vi "UtilityLib.Sixcolor.vi"(0 "State":T1 caption="index") -> (3 "booleanColor":u32(colorbox), 4 "elementBackground":u32(colorbox), 5 "elementText":u32(colorbox), 6 "elementTextWhite":u32(colorbox))   [LabVIEW 2014, in "UtilityLib.lvlib"]
doc: "By this VI five colors of a color box are defined by the \"State\":\n\n0 -> white (suggested meaning: no information available)\n1 -> darkgreen (suggested meaning: stand by/off)\n2 -> lightgreen (suggested meaning: on)\n3 -> yellow (suggested meaning: warning)\n4 -> red (suggested meaning: alarm/malfunction)\n5 -> black (suggested meaning: not implemented)\n6 -> blue (suggested meaning: user input/action required)\n7 -> pink (suggested meaning: important information, to be acknowledged)\n8-> system (system default color for GUI elements)\n9->control (default color for GUI control elements)\n10->indicator (default color for GUI indiciator elements)"
uses:
  UtilityLib.lvlib
  UtilityLib.valueStatus.ctl
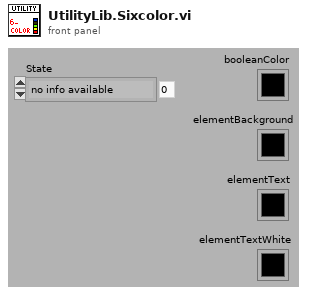
[diagram p1: front panel]
types:
  T1 = typedef "UtilityLib.lvlib/UtilityLib.valueStatus.ctl" = enum16{"no info available", "stand by/off", "on", "warning", "alarm/malfunction", "not implemented", "user action required", "important information", "system default", "control default", "indicator default", "button default"}
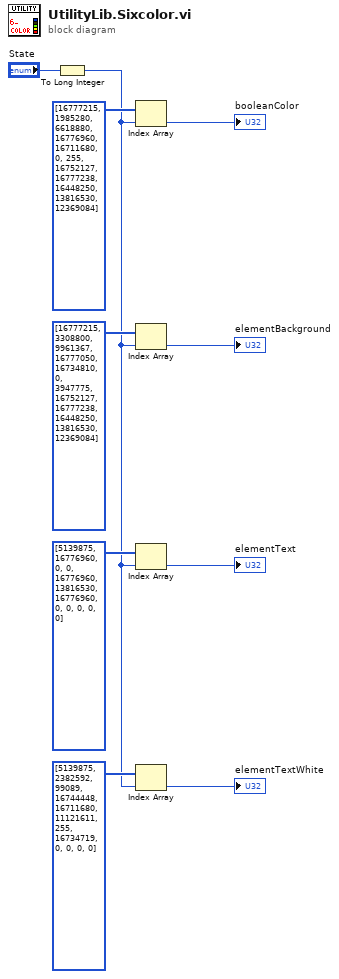
[diagram p0: block diagram]
diagram:
  n1 = To Long Integer(number="State") -> (32bit integer=w1:i32)
  n2 = Index Array(array=u32[] [16777215, 1985280, 6618880, 16776960, 16711680, 0, 255, 16752127, 16777238, 16448250, 13816530, 12369084], index=w1) -> (element=→"booleanColor":u32)
  n3 = Index Array(array=u32[] [16777215, 3308800, 9961367, 16777050, 16734810, 0, 3947775, 16752127, 16777238, 16448250, 13816530, 12369084], index=w1) -> (element=→"elementBackground":u32)
  n4 = Index Array(array=u32[] [5139875, 16776960, 0, 0, 16776960, 13816530, 16776960, 0, 0, 0, 0, 0], index=w1) -> (element=→"elementText":u32)
  n5 = Index Array(array=u32[] [5139875, 2382592, 99089, 16744448, 16711680, 11121611, 255, 16734719, 0, 0, 0, 0], index=w1) -> (element=→"elementTextWhite":u32)
